vi "Integrador (SubVI).vi"(1 "PID sale de rango":bool, 2 "Stop":bool, 4 "Ki":dbl, 5 "T":dbl, 6 "Error":dbl) -> (0 "Accion Integral":dbl)   [LabVIEW 2011]
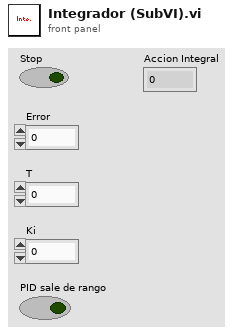
[diagram p1: front panel]
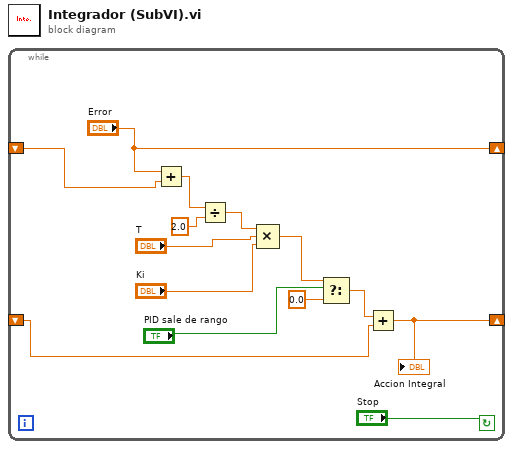
[diagram p0: block diagram]
diagram:
  n1 = while {
    shift-right: ["Error"] -> _
    shift-left: _ -> [w13]
    shift-right: [w3] -> _
    shift-left: _ -> [w2]
    stop <- "Stop" continue-if-true
    n2 = Add(x="Error", y=w13) -> (x+y=w12:dbl)
    n3 = Divide(x=w12, y=2.0) -> (x/y=w10:dbl)
    n4 = Compound Arithmetic op=MULTIPLY(w10, "T", "Ki") -> (w7:dbl)
    n5 = Select(t=w7, s="PID sale de rango", f=0.0) -> (s? t:f=w4:dbl)
    n6 = Add(x=w4, y=w2) -> (x+y=w3:dbl)
    "Accion Integral" <- w3
  }
